vi "niFPGA FFT Control Unit.vi"(0 "input valid":bool, 1 "Execution Constants":T1, 12 "ready for output":bool, 13 "reset":bool) -> (4 "enable fft":bool, 8 "control signals out":T2)   [LabVIEW 2017]
uses:
  <vilib>/rvi/Analysis/measure/FFT/templates/niFPGA FFT Control Signals.ctl
  <vilib>/rvi/Analysis/measure/FFT/templates/niFPGA FFT States.ctl
panel:
  in  "control signals type def":T2
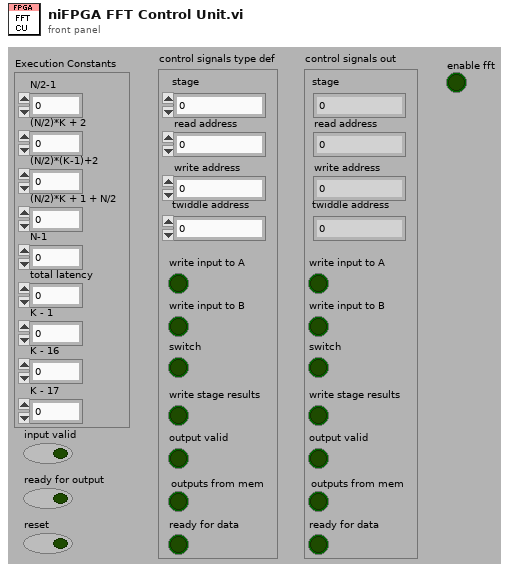
[diagram p1: front panel]
types:
  T1 = cluster{"N/2-1":u16, "(N/2)*K + 2":u16, "(N/2)*(K-1)+2":u16, "(N/2)*K + 1 + N/2":u16, "N-1":u16, "total latency":u16, "K - 1":u8, "K - 16":i8, "K - 17":i8}
  T2 = typedef "niFPGA FFT Control Signals.ctl" = cluster{"read address":u16, "switch":bool, "write input to B":bool, "write stage results":bool, "write input to A":bool, "output valid":bool, "twiddle address":u16, "write address":u16, "outputs from mem":bool, "ready for data":bool, "stage":u8}
  T3 = typedef "niFPGA FFT States.ctl" = enum8{"Input Only", "Transform", "Input/Output"}
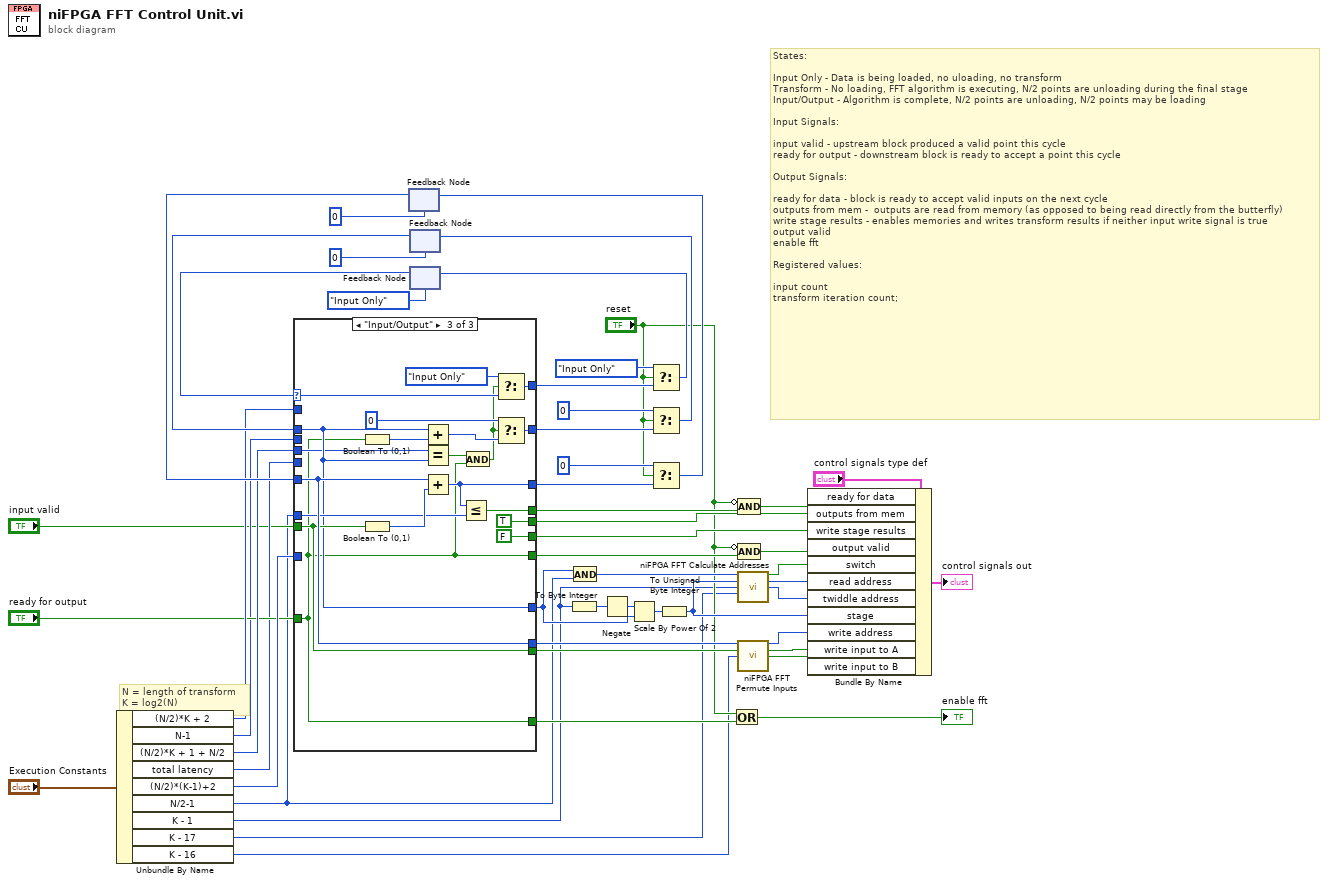
[diagram p0: block diagram]
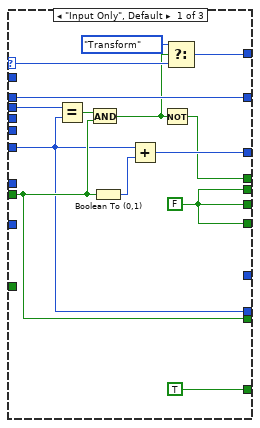
[diagram p2: hidden frame]
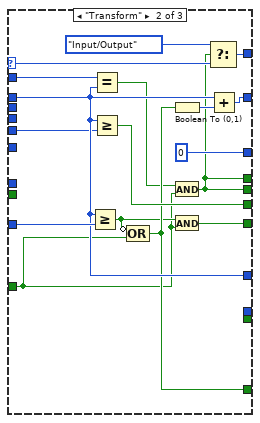
[diagram p3: hidden frame]
diagram:
  # "States:\n\nInput Only - Data is being loaded, no uloading, no transform\nTransform - No loading, FFT algorithm is executing, N/2 points are unloading during the final stage\nInput/Output - Algorithm is complete, N/2 points are unloading, N/2 points may be loading\n\nInput Signals:\n\ninput valid - upstream block produced a valid point this cycle\nready for output - downstream block is ready to accept a point this cycle\n\nOutput Signals:\n\nready for data - block is ready to accept valid inputs on the next cycle\noutputs from mem -  outputs are read from memory (as opposed to being read directly from the butterfly)\nwrite stage results - enables memories and writes transform results if neither input write signal is true\noutput valid\nenable fft\n\nRegistered values:\n\ninput count\ntransform iteration count;"
  # "N = length of transform\nK = log2(N)"
  n1 = Unbundle By Name("Execution Constants") -> ("(N/2)*K + 2"=w33:u16, "N-1"=w22:u16, "(N/2)*K + 1 + N/2"=w32:u16, "total latency"=w23:u16, "(N/2)*(K-1)+2"=w35:u16, "N/2-1"=w4:u16, "K - 1"=w3:u8, "K - 17"=w1:i8, "K - 16"=w2:i8)
  n2 = feedback #1(u16 0 ("t")) -> (w44:u16)
  n3 = feedback #2(u16 0 ("t")) -> (w34:u16)
  n4 = feedback #3(niFPGA_FFT_States."Input Only" ("Enum")) -> (w41:T3)
  n5 = case shown="\"Input/Output\"" w41 {
    selector: w41 -> [w64 w82 w103]
    tunnel: [w66 w81 w102] -> w48
    tunnel: w34 -> [w65 w76 w87]
    tunnel: [w65 w83 w100] -> w40
    tunnel: w44 -> [w59 _ w93]
    tunnel: "input valid" -> [w60 _ w88]
    tunnel: [w62 u16 0 w92] -> w38
    tunnel: [w55 w71 w84] -> w9
    tunnel: [w55 w79 FALSE] -> w47
    tunnel: [w60 _ w88] -> w21
    tunnel: [w59 _ w93] -> w20
    tunnel: [w55 w68 TRUE] -> w50
    tunnel: [_ w76 w87] -> w28
    tunnel: w33 -> [_ w77 _]
    tunnel: w35 -> [_ w78 _]
    tunnel: w32 -> [_ _ w85]
    tunnel: w22 -> [w58 _ _]
    tunnel: [w56 w68 w91] -> w11
    tunnel: "ready for output" -> [_ w67 w84]
    tunnel: [TRUE w74 w84] -> w5
    tunnel: w4 -> [_ _ w90]
    tunnel: w23 -> [_ w70 _]
    frame "Input Only", Default {
      w55 = FALSE
      n6 = Equal?(x=w58, y=w59) -> (x = y?=w61:bool)
      n7 = And(x=w61, y=w60) -> (x .and. y?=w57:bool)
      n8 = Boolean To (0,1)(Boolean=w60) -> (0, 1=w63:i16)
      n9 = Add(x=w59, y=w63) -> (x+y=w62:u16)
      n10 = Not(x=w57) -> (.not. x?=w56:bool)
      n11 = Select(t=niFPGA_FFT_States."Transform" ("Enum"), s=w57, f=w64) -> (s? t:f=w66:T3)
    }
    frame "Transform" {
      n12 = Greater Or Equal?(x=w76, y=w78) -> (x >= y?=w72:bool)
      n13 = Equal?(x=w77, y=w76) -> (x = y?=w73:bool)
      n14 = Greater Or Equal?(x=w76, y=w70) -> (x >= y?=w79:bool)
      n15 = Compound Arithmetic op=OR(invert w72, w67) -> (w74:bool)
      n16 = Boolean To (0,1)(Boolean=w74) -> (0, 1=w75:i16)
      n17 = And(x=w73, y=w67) -> (x .and. y?=w68:bool)
      n18 = And(x=w72, y=w67) -> (x .and. y?=w71:bool)
      n19 = Select(t=niFPGA_FFT_States."Input/Output" ("Enum"), s=w68, f=w82) -> (s? t:f=w81:T3)
      n20 = Add(x=w76, y=w75) -> (x+y=w83:u16)
    }
    frame "Input/Output" {
      n21 = Boolean To (0,1)(Boolean=w84) -> (0, 1=w95:i16)
      n22 = Boolean To (0,1)(Boolean=w88) -> (0, 1=w98:i16)
      n23 = Add(x=w87, y=w95) -> (x+y=w101:u16)
      n24 = Equal?(x=w85, y=w87) -> (x = y?=w86:bool)
      n25 = Add(x=w93, y=w98) -> (x+y=w92:u16)
      n26 = Less Or Equal?(x=w92, y=w90) -> (x <= y?=w91:bool)
      n27 = And(x=w86, y=w84) -> (x .and. y?=w94:bool)
      n28 = Select(t=niFPGA_FFT_States."Input Only" ("Enum"), s=w94, f=w103) -> (s? t:f=w102:T3)
      n29 = Select(t=u16 0, s=w94, f=w101) -> (s? t:f=w100:u16)
    }
  }
  n30 = To Byte Integer(number=w3) -> (8bit integer=w25:i8)
  n31 = And(x=w28, y=w4) -> (x .and. y?=w29:u16)
  n32 = Negate(x=w25) -> (-x=w27:i8)
  n33 = Scale By Power Of 2(n=w27, x=w28) -> (x*2^n=w26:u16)
  n34 = Select(t=niFPGA_FFT_States."Input Only" ("Enum"), s="reset", f=w48) -> (s? t:f=w45:T3)
  n35 = feedback-in #3(w45) -> ()
  n36 = Select(t=u16 0, s="reset", f=w40) -> (s? t:f=w42:u16)
  n37 = feedback-in #2(w42) -> ()
  n38 = Select(t=u16 0, s="reset", f=w38) -> (s? t:f=w43:u16)
  n39 = feedback-in #1(w43) -> ()
  n40 = To Unsigned Byte Integer(number=w26) -> (unsigned 8bit integer=w30:u8)
  n41 = Or(x="reset", y=w5) -> (x .or. y?=→"enable fft":bool)
  n42 = Compound Arithmetic op=AND(invert "reset", w11) -> (w10:bool)
  n43 = Compound Arithmetic op=AND(invert "reset", w9) -> (w8:bool)
  n44 = call <vilib>:"niFPGA FFT Calculate Addresses.vi"("butterfly count"=w29, "current stage"=w30, "K - 1"=w3, "K - 17"=w1) -> ("switch?"=w15:bool, "address"=w52:u16, "twiddle index"=w51:u16)  [unwired: 9 out]
  n45 = call <vilib>:"niFPGA FFT Permute Inputs.vi"("input index"=w20, "input valid"=w21, "K - 16"=w2) -> ("permuted index"=w18:u16, "write input to A"=w17:bool, "write input to B"=w16:bool)  [unwired: 10 out]
  n46 = Bundle By Name(cluster="control signals type def", "ready for data"=w10, "outputs from mem"=w50, "write stage results"=w47, "output valid"=w8, "switch"=w15, "read address"=w52, "twiddle address"=w51, "stage"=w30, "write address"=w18, "write input to A"=w17, "write input to B"=w16) -> (→"control signals out":T2)
